vi "Write to File.vi"(8 "error in (no error)":errorcluster, 11 "XML Report":refnum<class "XML Report.lvclass">) -> (0 "error out":errorcluster, 3 "XML Report out":refnum<class "XML Report.lvclass">)   [LabVIEW 2009, in "XML Report.lvclass"]
doc: "This dynamic dispatch VI takes the information in the object and writes it to a TXT file.\n\nAAL 9/09"
uses:
  XML Report.lvclass
  <vilib>/Utility/xml.llb/Write to XML File(string).vi
  Report Class/Report.lvclass
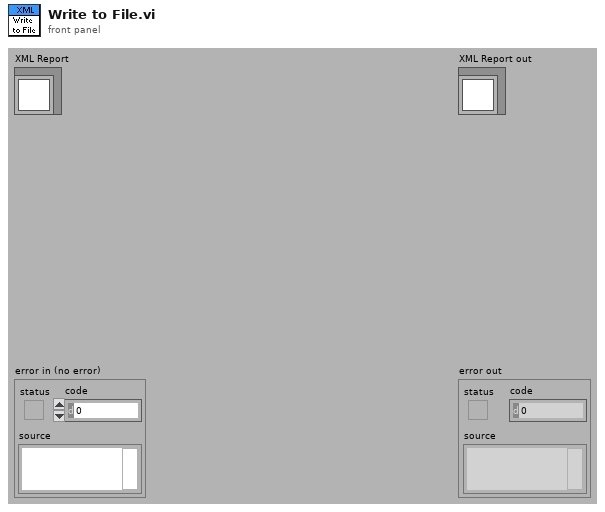
[diagram p1: front panel]
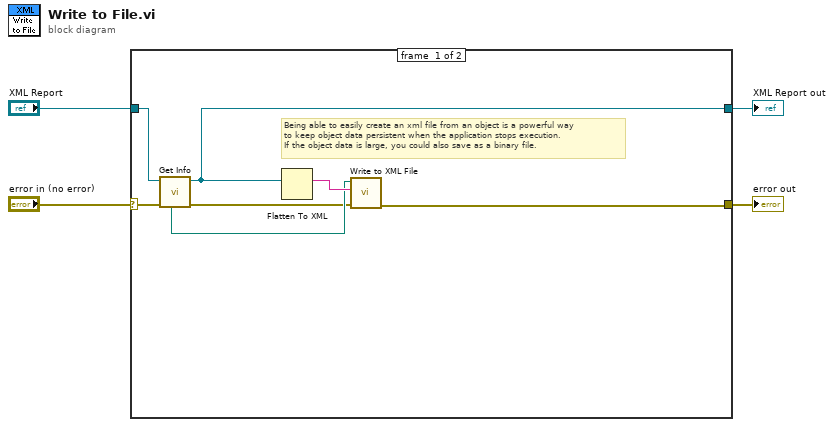
[diagram p0: block diagram]
diagram:
  n1 = case shown="No Error" "error in (no error)" {
    selector: "error in (no error)" -> [w10 w13]
    tunnel: [w5 w13] -> w3
    tunnel: [w9 w12] -> w1
    tunnel: "XML Report" -> [w11 w12]
    frame #0 {
      # "Being able to easily create an xml file from an object is a powerful way \nto keep object data persistent when the application stops execution.  \nIf the object data is large, you could also save as a binary file."
      n2 = call "Get Info.vi"("error in (no error)"=w10, "Report"=w11) -> ("error out"=w6:errorcluster, "Report out"=w9:refnum<class "XML Report.lvclass">, "Path"=w7:path)  [unwired: 7 out]
      n3 = Flatten To XML(anything=w9) -> (xml string=w8:string)
      n4 = call-poly <vilib>:"Write to XML File.vi"("error in (no error)"=w6, "XML Input"=w8, "XML File Path"=w7) -> ("error out"=w5:errorcluster)  [unwired: 2 in, 6 out]
    }
    frame #1 {
    }
  }
  "error out" <- w3
  "XML Report out" <- w1
